vi "Send unsent changes.vi"(0 "Fiber Auto Collimation state data in":refnum<class "Fiber Auto Collimation state data.lvclass">) -> (2 "Fiber Auto Collimation state data out":refnum<class "Fiber Auto Collimation state data.lvclass">)   [LabVIEW 2018, in "Fiber Auto Collimation state data.lvclass"]
doc: "If there are any elements of the state data that have been marked as \"changed\", this VI sends an event notification so that the UI will update to show those changes. After sending the event, the change list is cleared.\n\nThis VI is present at the end of each case in the main controller loop, but can be added during the loop as well if the changes made need to be updated sooner and the changes are unconditional (i.e. the wire doesn't branch in a way that means that a different wire might make it out of the case instead of the one this VI was on)."
uses:
  Fiber Auto Collimation state data.lvclass
  Fiber Auto Collimation state data.lvclass/Fiber Auto Collimation state data.ctl
  <vilib>/event_ctls.llb/usereventprio.ctl
  <vilib>/Utility/error.llb/Clear Errors.vi
  <userlib>/nLight Error Handling/Log any errors.vi
  References/Fiber Auto Collimation References.lvclass
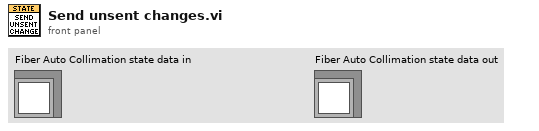
[diagram p1: front panel]
types:
  T1 = typedef "Fiber Auto Collimation state data.lvclass/Tracked state data.ctl" = enum16{"No update", "Permission level", "Username", "Test running", "DUT Serial", "Test status", "MOM Lot", "Loaded test recipe", "Model case running", "Station status", "BV data", "Defect Identify data", "Axis Position data", "Fiber Ass PN", "Operator", "RunTime", "VBAI", "Steps Cycle Time"}
  T2 = typedef "usereventprio.ctl" = enum32{"high priority", "normal priority"}
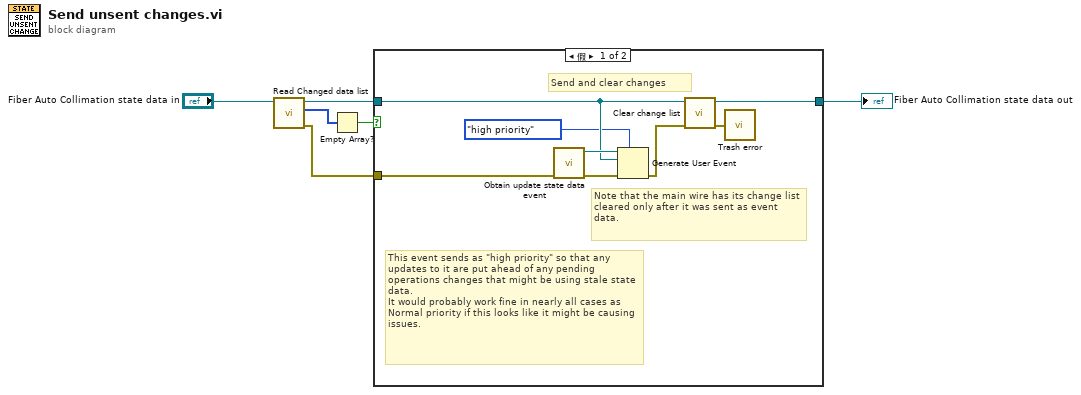
[diagram p0: block diagram]
diagram:
  n1 = call "Read Changed data list.vi"("Fiber Auto Collimation state data in"="Fiber Auto Collimation state data in") -> ("error out"=w1:errorcluster, "Changed data list"=w4:T1[], "Fiber Auto Collimation state data out"=w5:refnum<class "Fiber Auto Collimation state data.lvclass">)  [unwired: 8 in]
  n2 = Empty Array?(array=w4) -> (empty?=w3:bool)
  n3 = case shown="假" w3 {
    tunnel: [w14 w15] -> w6
    tunnel: w5 -> [w11 w15]
    tunnel: w1 -> [w8 _]
    frame False {
      # "This event sends as \"high priority\" so that any updates to it are put ahead of any pending operations changes that might be using stale state data.\nIt would probably work fine in nearly all cases as Normal priority if this looks like it might be causing issues."
      # "Note that the main wire has its change list cleared only after it was sent as event data."
      # "Send and clear changes"
      n4 = call "Obtain update state data event.vi"("error in (no error)"=w8) -> ("error out"=w13:errorcluster, "Update state data"=w12:refnum<user-event>)  [unwired: 9 in]
      n5 = Generate User Event(priority (normal)=usereventprio."high priority", user event=w12, event data cluster=w11, error in=w13) -> (error out=w9:errorcluster)  [unwired: 1 out]
      n6 = call "Clear change list.vi"("error in (no error)"=w9, "Fiber Auto Collimation state data in"=w11) -> ("error out"=w7:errorcluster, "Fiber Auto Collimation state data out"=w14:refnum<class "Fiber Auto Collimation state data.lvclass">)  [unwired: 8 in]
      n7 = call <userlib>:"Trash error.vi"("error in"=w7) -> ()  [unwired: 15 in]
    }
    frame True {
      # "No changes logged, do nothing"
    }
  }
  "Fiber Auto Collimation state data out" <- w6
